vi "Get VI Reference.vi"(8 "error in (no error)":errorcluster, 10 "VI name":string, 11 "Test Finder":refnum<class "Test Finder.lvclass">) -> (0 "error out":errorcluster, 1 "Found?":bool, 2 "Reference":refnum<vi>, 3 "Test Finder out":refnum<class "Test Finder.lvclass">)   [LabVIEW 2020, in "Test Finder.lvclass"]
uses:
  Helper Classes/Test Finder/Test Finder.lvclass
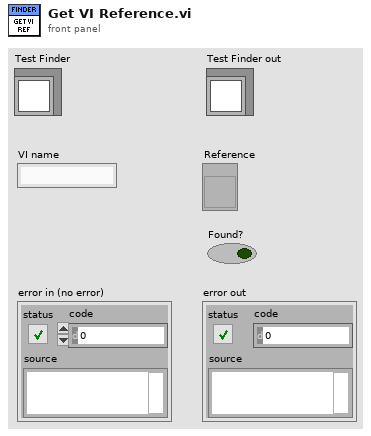
[diagram p1: front panel]
types:
  T1 = map{string, cluster{"Dynamic Methods":map{string, path}, "Static Methods":map{string, path}}}
  T2 = cluster{"Dynamic Methods":map{string, path}, "Static Methods":map{string, path}}
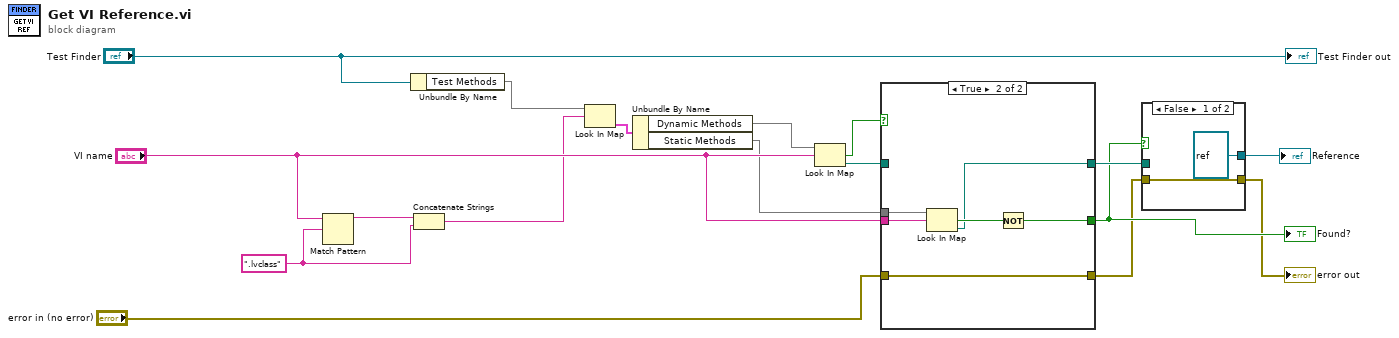
[diagram p0: block diagram]
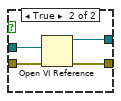
[diagram p2: hidden frame]
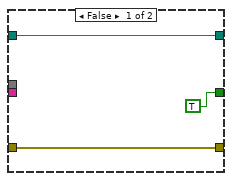
[diagram p3: hidden frame]
diagram:
  w12 = ".lvclass" ("regular expression")
  n1 = Match Pattern(string="VI name", regular expression=w12) -> (before substring=w13:string)  [unwired: 1 in, 3 out]
  n2 = Unbundle By Name("Test Finder") -> ("Test Methods"=w14:T1)
  n3 = Concatenate Strings(w13, w12) -> (w8:string)
  n4 = Look In Map(map=w14, key=w8) -> (value=w11:T2)  [unwired: 1 in, 1 out]
  n5 = Unbundle By Name(w11) -> ("Dynamic Methods"=w7:map{string, path}, "Static Methods"=w6:map{string, path})
  n6 = Look In Map(map=w7, key="VI name") -> (key not found?=w9:bool, value=w10:path)  [unwired: 1 in]
  n7 = case shown="True" w9 {
    tunnel: w10 -> [w18 _]
    tunnel: "error in (no error)" -> [w20 w22]
    tunnel: [w20 w22] -> w2
    tunnel: [TRUE w23] -> w4
    tunnel: w6 -> [_ w26]
    tunnel: "VI name" -> [_ w25]
    tunnel: [w18 w21] -> w5
    frame False {
    }
    frame True {
      n8 = Look In Map(map=w26, key=w25) -> (key not found?=w24:bool, value=w21:path)  [unwired: 1 in]
      n9 = Not(x=w24) -> (.not. x?=w23:bool)
    }
  }
  "Found?" <- w4
  n10 = case shown="False" w4 {
    tunnel: w5 -> [_ w32]
    tunnel: w2 -> [w28 w31]
    tunnel: [w28 w30] -> w3
    tunnel: [refnum<vi> refnum ("vi reference") w29] -> w1
    frame False {
    }
    frame True {
      n11 = Open VI Reference(vi path=w32, error in (no error)=w31) -> (vi reference=w29:refnum<vi>, error out=w30:errorcluster)  [unwired: 4 in]
    }
  }
  "error out" <- w3
  "Reference" <- w1
  "Test Finder out" <- "Test Finder"
